vi "测试-数据库关键字搜索.vi"() -> ()   [LabVIEW 2022 SP3]
uses:
  <vilib>/addons/database/Connection.llb/DB Tools Open Connec (String).vi
  <vilib>/addons/database/Connection.llb/Conn Execute.vi
  <vilib>/addons/database/Recordset.llb/Rec Fetch Recordset Data (R).vi
  <vilib>/addons/database/Recordset.llb/Rec Destroy - Connection.vi
  <vilib>/addons/database/_DB Variant To Data/Database Variant To Data.xnode
  <vilib>/addons/database/NI_Database_API.lvlib
panel:
  in  "关键字":string
  in  "表名":string
  out "data":string[][](array[string])
  in  "路径":path
  out "error out":errorcluster
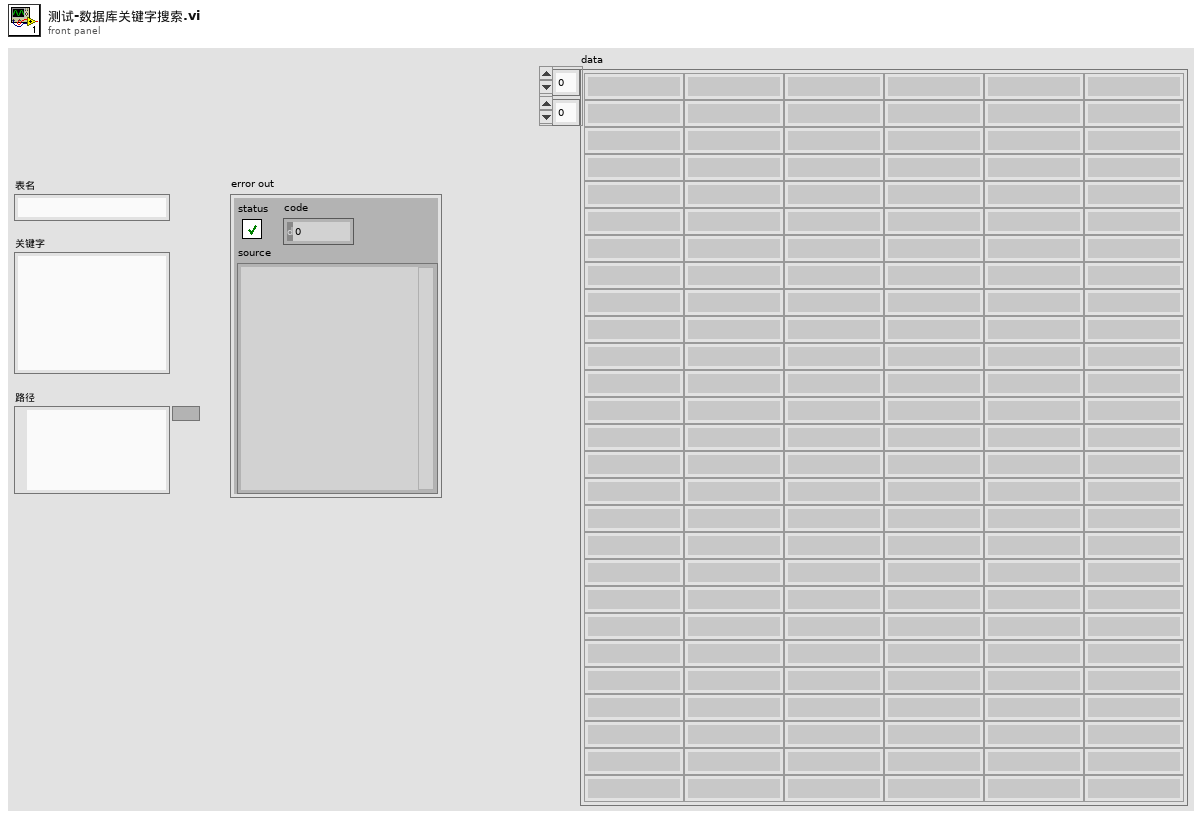
[diagram p1: front panel]
types:
  T1 = typedef "NI_Database_API.lvlib/Conn ObjectReference.ctl" = refnum<k1>
  T2 = typedef "NI_Database_API.lvlib/Rec ObjectReference.ctl" = refnum<k1>
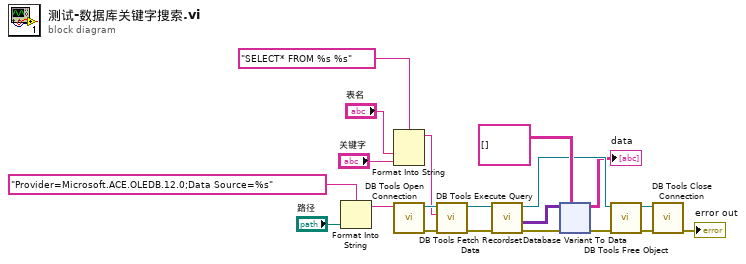
[diagram p0: block diagram]
diagram:
  n1 = Format Into String(format string="Provider=Microsoft.ACE.OLEDB.12.0;Data Source=%s" ("格式字符串"), "路径") -> (resulting string=w13:string)  [unwired: 2 in, 1 out]
  n2 = Format Into String(format string="SELECT* FROM %s %s" ("格式字符串"), "表名", "关键字") -> (resulting string=w1:string)  [unwired: 2 in, 1 out]
  n3 = call-poly <vilib>:"DB Tools Open Connection.vi"("connection information"=w13) -> ("error out"=w6:errorcluster, "connection reference"=w7:T1)  [unwired: 7 in]
  n4 = call-poly <vilib>:"DB Tools Execute Query.vi"("error in (no error)"=w6, "SQL query"=w1, "connection reference"=w7) -> ("error out"=w19:errorcluster, "recordset reference"=w10:T2)  [unwired: 5 in]
  n5 = call-poly <vilib>:"DB Tools Fetch Recordset Data.vi"("error in (no error)"=w19, "recordset reference"=w10) -> ("error out"=w20:errorcluster, "recordset data"=w11:variant[][], "recordset reference out"=w9:T2)  [unwired: 3 in]
  n6 = xnode "Database Variant To Data"("database variant"=w11, "error in (no error)"=w20, "type"=string[][] []) -> ("data"=→"data":string[][], "error out"=w18:errorcluster)
  n7 = call-poly <vilib>:"DB Tools Free Object.vi"("error in (no error)"=w18, "recordset reference"=w9) -> ("error out"=w17:errorcluster, "connection reference"=w8:T1)  [unwired: 8 in]
  n8 = call <vilib>:"DB Tools Close Connection.vi"("error in (no error)"=w17, "connection reference"=w8) -> ("error out"=→"error out":errorcluster)  [unwired: 5 in]
